vi "SNMP GET VALUES.vi"(0 "IP Address":string, 1 "Community":string, 2 "Timeout":i32, 7 "error in":errorcluster, 16 "OIDs":string[](array[string])) -> (13 "error snmp":bool, 14 "result":dbl[](array[numeric]), 15 "Vac_input3":dbl, 17 "Vac_input2":dbl, 18 "Ibat":dbl, 19 "Vac_input1":dbl, 20 "Pot_panel_out":dbl, 21 "I_Load_Inv_R":dbl, 22 "I_Load_Inv_S":dbl, 23 "I_Load_Inv_T":dbl, 24 "Pot_load_out":dbl, 25 "Nivel_bat_out":dbl, 26 "Ubat":dbl, 27 "error out":errorcluster)   [LabVIEW 2015]
uses:
  Login Window Control Folder/global variable.vi
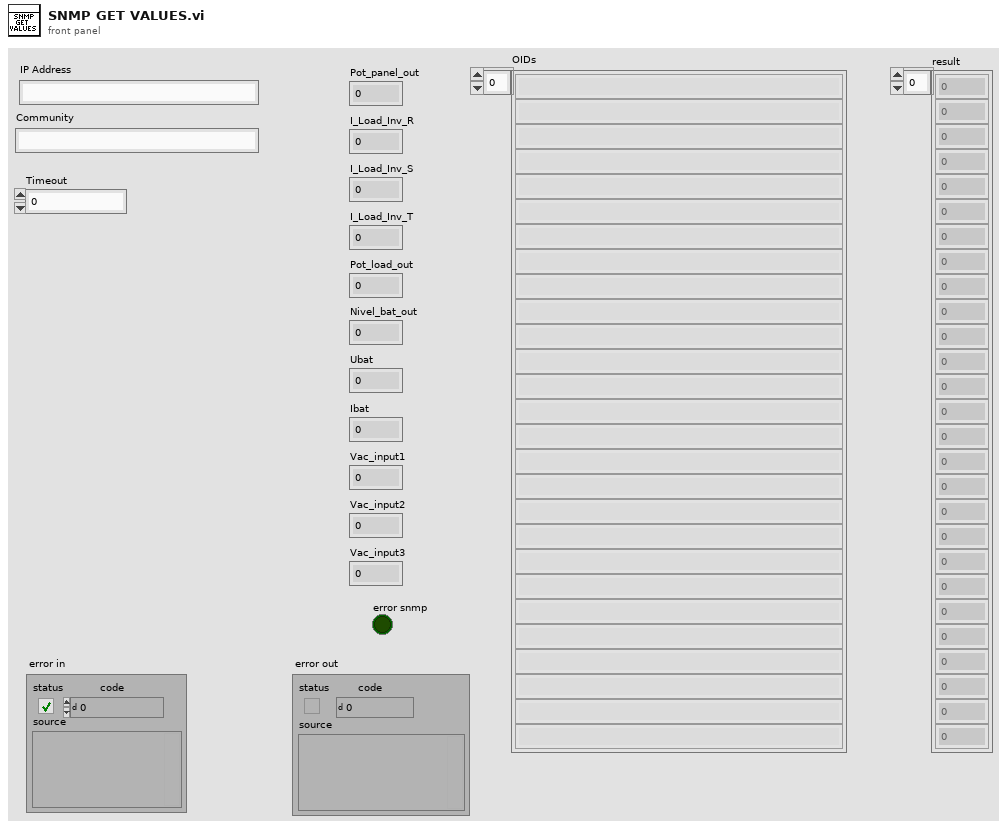
[diagram p1: front panel]
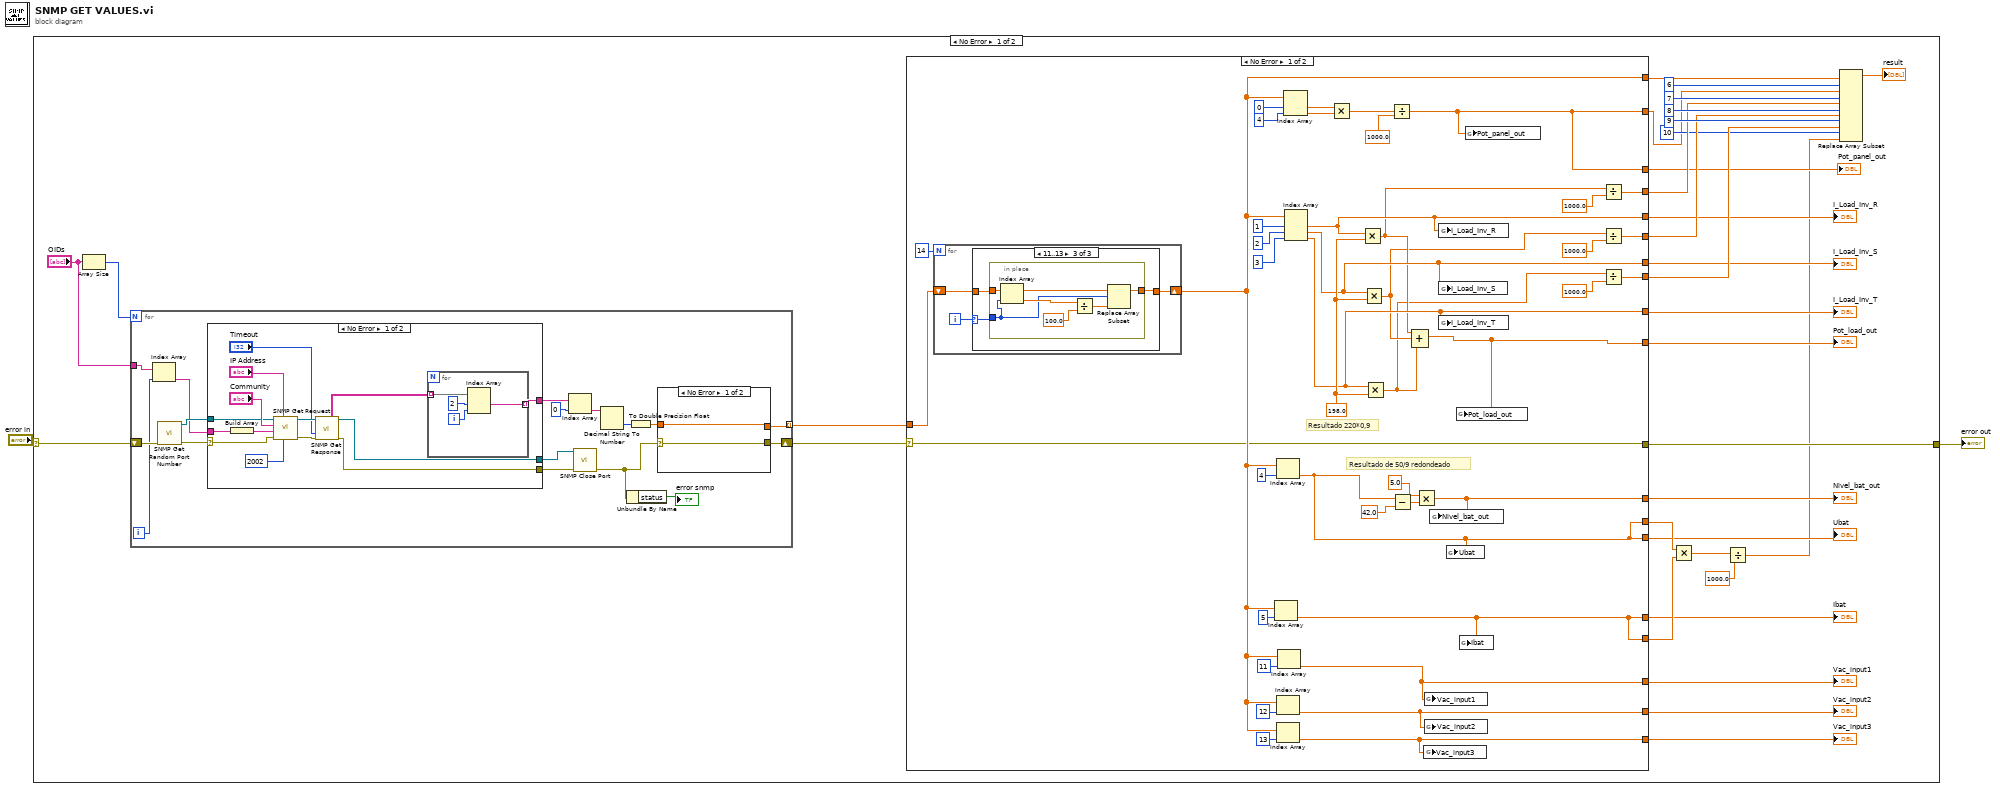
[diagram p0: block diagram]
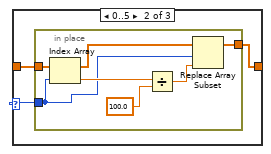
[diagram p3: hidden frame]
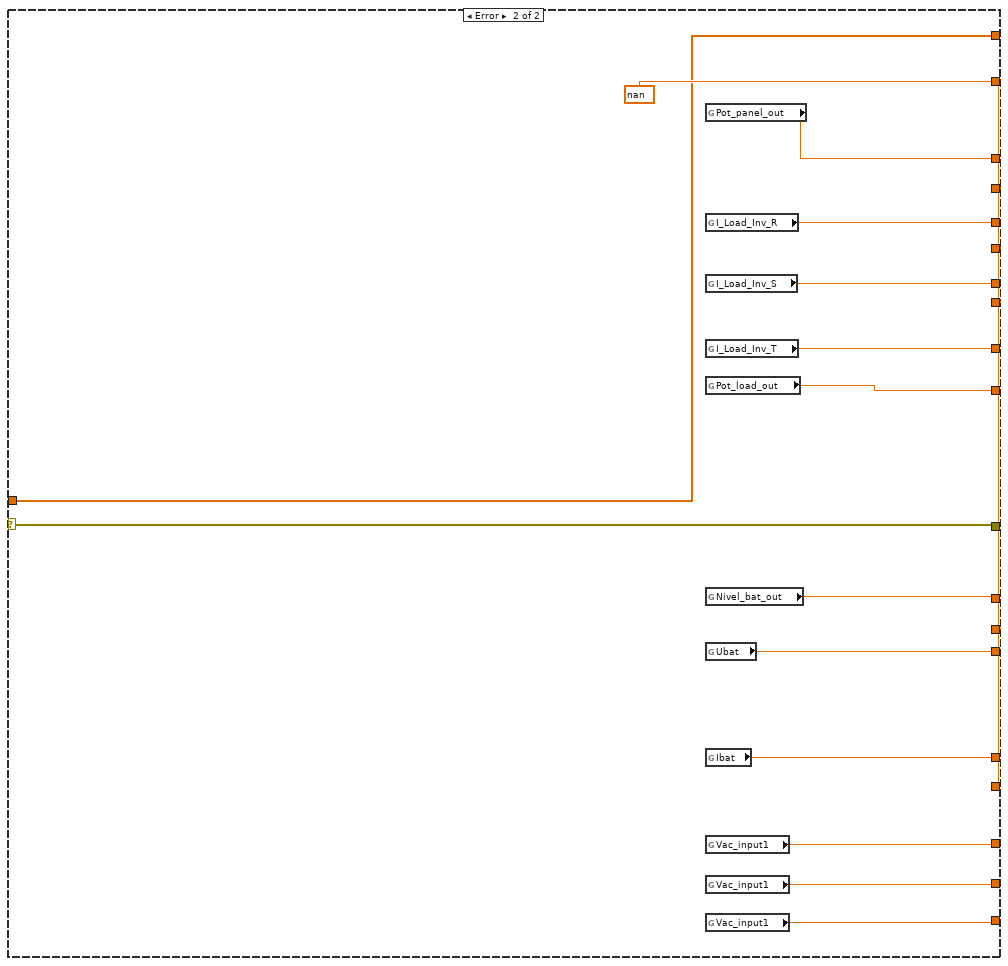
[diagram p4: hidden frame]
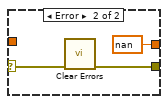
[diagram p5: hidden frame]
diagram:
  n1 = case shown="No Error" "error in" {
    selector: "error in" -> [w7 w156]
    tunnel: [w8 w156] -> w1
    frame No Error {
      n2 = Array Size(array="OIDs") -> (size(s)=w35:i32)
      n3 = for {
        N: w35 -> [_]
        tunnel: "OIDs" -> [w116]
        tunnel: [w123] -> w6 mode=indexing
        shift-right: [w121] -> w9
        shift-left: w7 -> [w117]
        i -> [w114]
        n4 = Index Array(array=w116, index=w114) -> (element=w115:string)
        n5 = call "SNMP Get Random Port Number.vi"("error in (no error)"=w117) -> ("error out"=w122:errorcluster, "connection ID"=w118:refnum<k16>)  [unwired: 8 in, 1 out]
        n6 = case shown="No Error" w122 {
          selector: w122 -> [w138 w154]
          tunnel: w118 -> [w139 w155]
          tunnel: [w145 w155] -> w130
          tunnel: [w144 w154] -> w129
          tunnel: w115 -> [w142 _]
          tunnel: [w137 _] -> w128
          frame No Error {
            n7 = Build Array(w142) -> (w141:string[])
            n8 = call "SNMP Get Request.vi"("UDP Port"=u16 2002, "IP Address"="IP Address", "error in (no error)"=w138, "OID ARRAY"=w141, "Community Name"="Community", "connection ID"=w139) -> ("error out"=w146:errorcluster, "connection ID"=w147:refnum<k16>)  [unwired: 3 in, 1 out]
            n9 = call "SNMP Get Response.vi"("connection ID"=w147, "timeout ms (25000)"="Timeout", "error in (no error)"=w146) -> ("SnmpDataAsStrings"=w143:string[][], "connection ID out"=w145:refnum<k16>, "error out"=w144:errorcluster)  [unwired: 4 in, 6 out]
            n10 = for {
              tunnel: w143 -> [w153] mode=indexing
              tunnel: [w150] -> w137 mode=indexing
              i -> [w152]
              n11 = Index Array(array=w153, index #1=2 ("index"), index #2=w152) -> (element #1=w150:string)  [unwired: 1 out]
            }
          }
          frame Error {
          }
        }
        n12 = Index Array(array=w128, index=0) -> (element=w126:string)
        n13 = call "SNMP Close Port.vi"("error in (no error)"=w129, "connection ID"=w130) -> ("error out"=w120:errorcluster)  [unwired: 8 in, 1 out]
        n14 = Decimal String To Number(string=w126) -> (number=w125:i32)  [unwired: 2 in, 1 out]
        n15 = Unbundle By Name(w120) -> ("status"=→"error snmp":bool)
        n16 = To Double Precision Float(number=w125) -> (double precision float=w124:dbl)
        n17 = case shown="No Error" w120 {
          selector: w120 -> [w132 w135]
          tunnel: [w132 w134] -> w121
          tunnel: w124 -> [w131 _]
          tunnel: [w131 nan] -> w123
          frame No Error {
          }
          frame Error {
            n18 = call <vilib>:"Clear Errors.vi"("error in (no error)"=w135) -> ("error out"=w134:errorcluster)  [unwired: 5 in, 1 out]
          }
        }
      }
      n19 = case shown="No Error" w9 {
        selector: w9 -> [w52 w101]
        tunnel: [w46 w105] -> w10
        tunnel: [w44 w105] -> w29
        tunnel: [w41 w105] -> w28
        tunnel: [w37 w105] -> w27
        tunnel: [w36 w110] -> w21
        tunnel: [w59 w106] -> w15
        tunnel: [w66 w108] -> w17
        tunnel: [w60 w107] -> w16
        tunnel: [w63 w113] -> w14
        tunnel: [w61 w112] -> w13
        tunnel: [w62 w111] -> w12
        tunnel: [w46 w109] -> w22
        tunnel: [w60 w105] -> w25
        tunnel: [w59 w105] -> w24
        tunnel: [w58 w104] -> w20
        tunnel: [w57 w103] -> w19
        tunnel: [w56 w102] -> w18
        tunnel: w6 -> [w54 w100]
        tunnel: [w53 w100] -> w11
        tunnel: [w52 w101] -> w8
        frame No Error {
          w73 = 198.0 ("y")
          # "Resultado 220*0,9"
          # "Resultado de 50/9 redondeado"
          n20 = for {
            N: 14 -> [_]
            shift-right: [w79] -> w53
            shift-left: w54 -> [w80]
            i -> [w78]
            n21 = case shown="11..13" w78 {
              selector: w78 -> [_ w82 w91]
              tunnel: w80 -> [w81 w84 w93]
              tunnel: [w81 w83 w92] -> w79
              frame Default {
              }
              frame 0..5 {
                n22 = in-place {
                  in-place-border: w82 -> [w85]
                  in-place-border: w84 -> [w87]
                  in-place-border: [w88] -> w83
                  n23 = Index Array(array=w87, index=w85) -> (element=w90:dbl)
                  n24 = Divide(x=w90, y=100.0) -> (x/y=w86:dbl)
                  n25 = Replace Array Subset(array=w87, new element=w86, index=w85) -> (w88:dbl[])
                }
              }
              frame 11..13 {
                n26 = in-place {
                  in-place-border: w91 -> [w94]
                  in-place-border: w93 -> [w95]
                  in-place-border: [w96] -> w92
                  n27 = Index Array(array=w95, index=w94) -> (element=w99:dbl)
                  n28 = Divide(x=w99, y=100.0) -> (x/y=w97:dbl)
                  n29 = Replace Array Subset(array=w95, new element=w97, index=w94) -> (w96:dbl[])
                }
              }
            }
          }
          n30 = Index Array(array=w53, index=5) -> (element=w59:dbl)
          n31 = Index Array(array=w53, index=4) -> (element=w60:dbl)
          n32 = Index Array(array=w53, index=12) -> (element=w61:dbl)
          n33 = Index Array(array=w53, index=13) -> (element=w62:dbl)
          n34 = Index Array(array=w53, index=11) -> (element=w63:dbl)
          n35 = Index Array(array=w53, index #1=0 ("index"), index #2=4 ("index")) -> (element #1=w76:dbl, element #2=w77:dbl)
          n36 = Index Array(array=w53, index #1=1 ("index"), index #2=2 ("index"), index #3=3 ("index")) -> (element #1=w58:dbl, element #2=w57:dbl, element #3=w56:dbl)
          n37 = Multiply(x=w76, y=w77) -> (x*y=w47:dbl)
          n38 = Multiply(x=w58, y=w73) -> (x*y=w43:dbl)
          n39 = Multiply(x=w57, y=w73) -> (x*y=w40:dbl)
          n40 = Multiply(x=w56, y=w73) -> (x*y=w38:dbl)
          n41 = Divide(x=w47, y=1000.0) -> (x/y=w46:dbl)
          n42 = Subtract(x=w60, y=42.0) -> (x-y=w69:dbl)
          n43 = Compound Arithmetic op=ADD(w43, w40, w38) -> (w36:dbl)
          n44 = Multiply(x=5.0, y=w69) -> (x*y=w66:dbl)
          n45 = global write "global variable.vi" "Vac_input3"(w62) -> ()
          n46 = global write "global variable.vi" "Vac_input1"(w63) -> ()
          n47 = global write "global variable.vi" "Vac_input2"(w61) -> ()
          n48 = global write "global variable.vi" "Nivel_bat_out"(w66) -> ()
          n49 = global write "global variable.vi" "I_Load_Inv_R"(w58) -> ()
          n50 = global write "global variable.vi" "I_Load_Inv_S"(w57) -> ()
          n51 = global write "global variable.vi" "I_Load_Inv_T"(w56) -> ()
          n52 = global write "global variable.vi" "Ubat"(w60) -> ()
          n53 = global write "global variable.vi" "Pot_load_out"(w36) -> ()
          n54 = global write "global variable.vi" "Ibat"(w59) -> ()
          n55 = global write "global variable.vi" "Pot_panel_out"(w46) -> ()
          n56 = Divide(x=w43, y=1000.0) -> (x/y=w44:dbl)
          n57 = Divide(x=w40, y=1000.0) -> (x/y=w41:dbl)
          n58 = Divide(x=w38, y=1000.0) -> (x/y=w37:dbl)
        }
        frame Error {
          w105 = nan
          n59 = global read "global variable.vi" "Pot_panel_out"() -> (w109:dbl)
          n60 = global read "global variable.vi" "I_Load_Inv_R"() -> (w104:dbl)
          n61 = global read "global variable.vi" "I_Load_Inv_S"() -> (w103:dbl)
          n62 = global read "global variable.vi" "I_Load_Inv_T"() -> (w102:dbl)
          n63 = global read "global variable.vi" "Pot_load_out"() -> (w110:dbl)
          n64 = global read "global variable.vi" "Nivel_bat_out"() -> (w108:dbl)
          n65 = global read "global variable.vi" "Ubat"() -> (w107:dbl)
          n66 = global read "global variable.vi" "Ibat"() -> (w106:dbl)
          n67 = global read "global variable.vi" "Vac_input1"() -> (w113:dbl)
          n68 = global read "global variable.vi" "Vac_input1"() -> (w112:dbl)
          n69 = global read "global variable.vi" "Vac_input1"() -> (w111:dbl)
        }
      }
      "Pot_panel_out" <- w22
      "Pot_load_out" <- w21
      "I_Load_Inv_R" <- w20
      "I_Load_Inv_S" <- w19
      "I_Load_Inv_T" <- w18
      "Nivel_bat_out" <- w17
      "Ubat" <- w16
      "Ibat" <- w15
      "Vac_input1" <- w14
      "Vac_input2" <- w13
      "Vac_input3" <- w12
      n70 = Multiply(x=w25, y=w24) -> (x*y=w4:dbl)
      n71 = Divide(x=w4, y=1000.0) -> (x/y=w3:dbl)
      n72 = Replace Array Subset(array=w11, new element #1=w10, index #1=6 ("index"), new element #2=w29, index #2=7 ("index"), new element #3=w28, index #3=8 ("index"), new element #4=w27, index #4=9 ("index"), new element #5=w3, index #5=10 ("index")) -> (→"result":dbl[])
    }
    frame Error {
    }
  }
  "error out" <- w1
